vi "Control Page.vi"(8 "?":errorcluster) -> ()   [LabVIEW 2023, in "Vires VTD System Explorer.lvlib"]
uses:
  Vires VTD System Explorer.lvlib
  <vilib>/NI VeriStand/Custom Device API/Custom Device Item Ref.ctl
  <vilib>/NI VeriStand/Custom Device API/Custom Device API.lvlib
panel:
  in  "Header":cluster{"Section Name":string}={"Section Name"="Custom Device Item Settings"}
  in  "Description":string
  in  "Name":string
  in  "Node Ptr":T1 format="%.0x"
  out "error out":errorcluster
  in  "SHDocVw.IWebBrowser2":refnum<k7>(container)
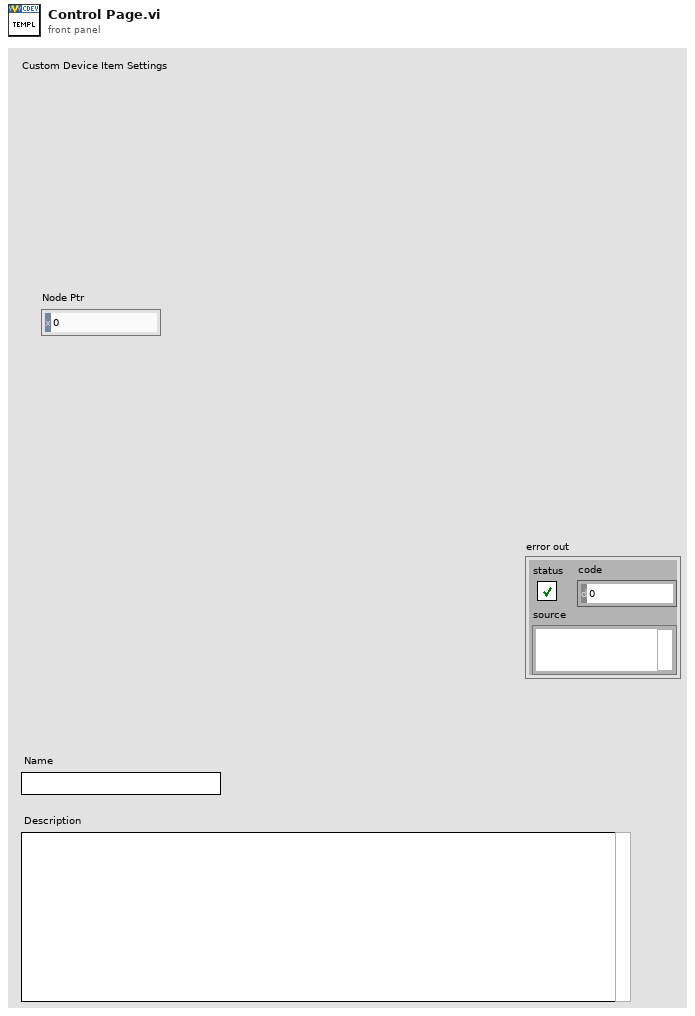
[diagram p1: front panel]
types:
  T1 = typedef "Custom Device API.lvlib/Custom Device Item Ref.ctl" = u64
  T2 = typedef "Custom Device API.lvlib/Custom Device Item Info.ctl" = cluster{"Name":string, "Is Channel":bool, "GUID":string, "Is Waveform":bool}
  T3 = typedef "Custom Device API.lvlib/Custom Device Commands.ctl" = enum16{"Default", "Item renamed", "Shutdown", "Dynamic button pressed"}
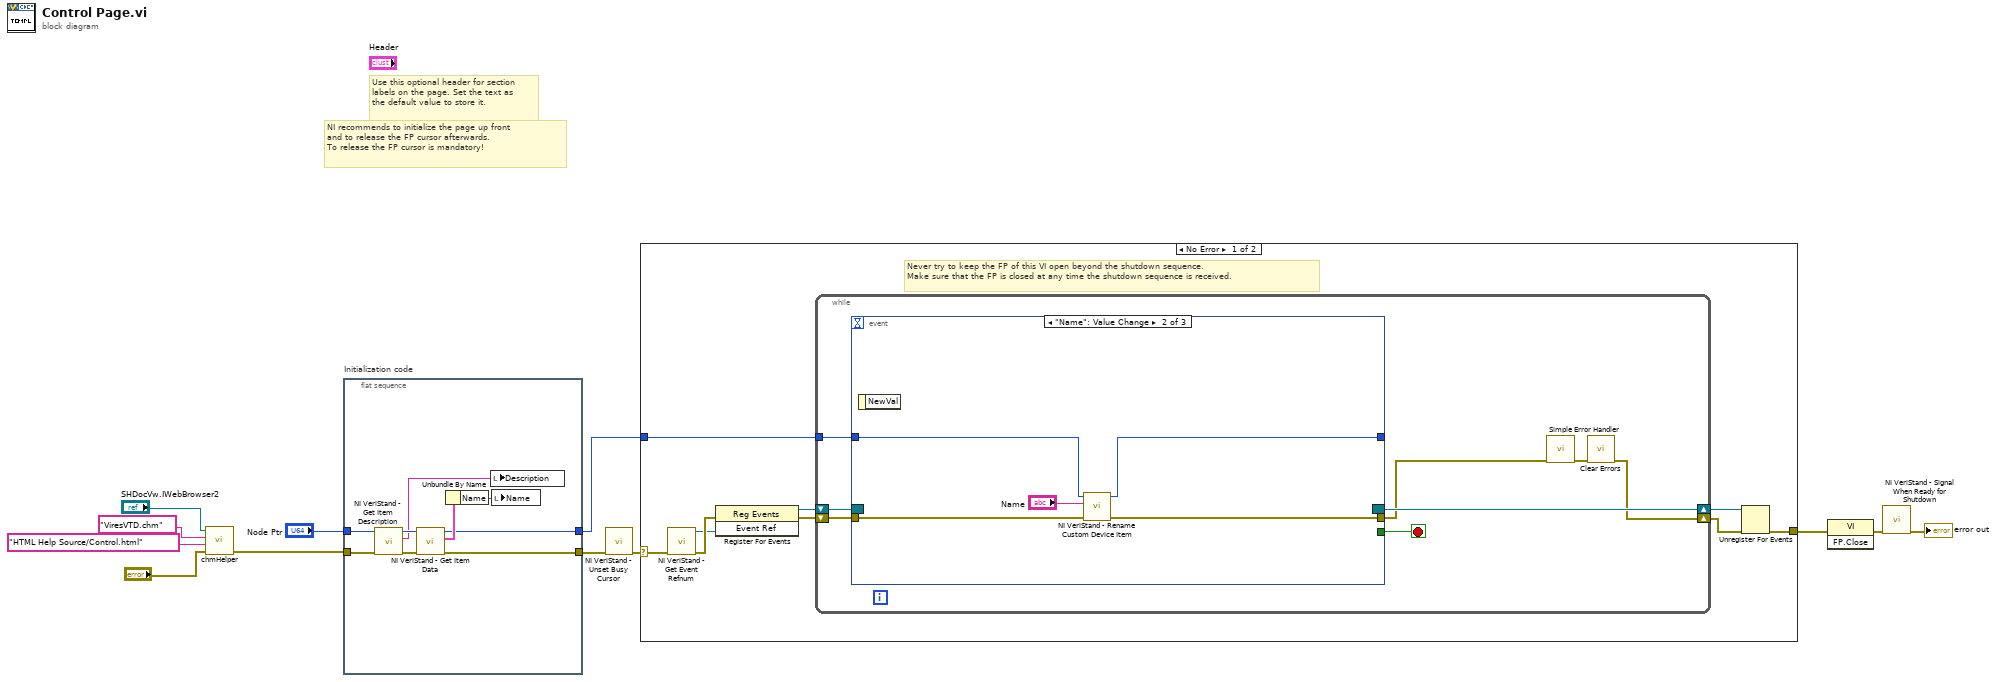
[diagram p0: block diagram]
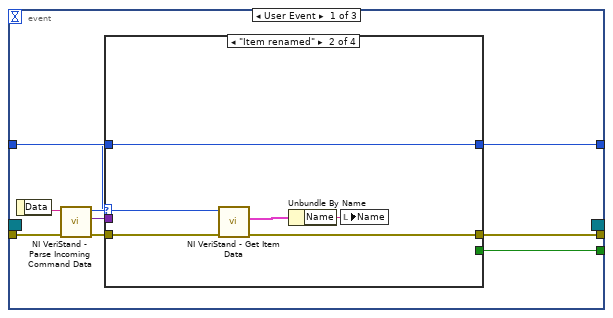
[diagram p2: hidden frame]
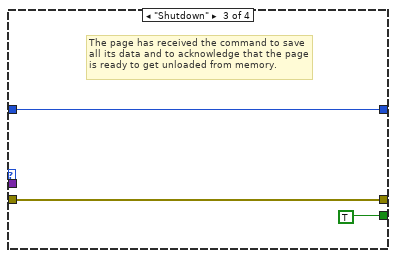
[diagram p4: hidden frame]
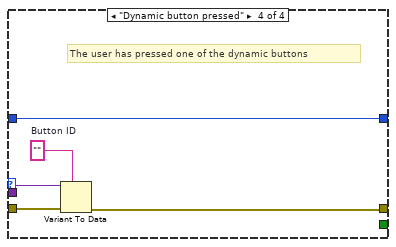
[diagram p5: hidden frame]
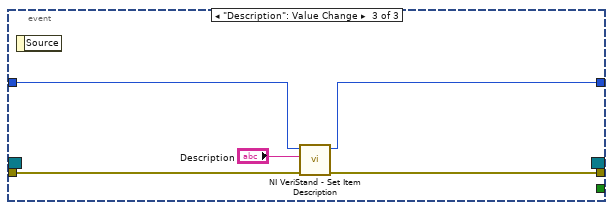
[diagram p6: hidden frame]
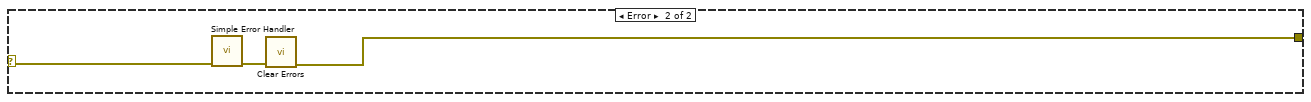
[diagram p7: hidden frame]
diagram:
  # "Use this optional header for section labels on the page. Set the text as the default value to store it."
  # "NI recommends to initialize the page up front\nand to release the FP cursor afterwards.\nTo release the FP cursor is mandatory!"
  n1 = call "chmHelper.vi"("error in (no error)"="?", "HTML File"="HTML Help Source/Control.html", "Main CHM File"="ViresVTD.chm" ("HTML File"), "Automation Refnum in"="SHDocVw.IWebBrowser2") -> ("error out"=w1:errorcluster)  [unwired: 7 in]
  n2 = flat-sequence "Initialization code" {
    tunnel: w1 -> [w20]
    tunnel: "Node Ptr" -> [w19]
    tunnel: [w14] -> w4
    tunnel: [w13] -> w2
    frame #0 {
      n3 = call <vilib>:"NI VeriStand - Get Item Description.vi"("error in (no error)"=w20, "Item Ref in"=w19) -> ("error out"=w17:errorcluster, "Description"=w18:string, "Item Ref out"=w21:T1)  [unwired: 7 out]
      n4 = call <vilib>:"NI VeriStand - Get Item Data.vi"("error in (no error)"=w17, "Item Ref in"=w21) -> ("error out"=w14:errorcluster, "Item Info"=w16:T2, "Item Ref out"=w13:T1)  [unwired: 7 out]
      n5 = Unbundle By Name(w16) -> ("Name"=w15:string)
      n6 = local write "Description"(w18) -> ()
      n7 = local write "Name"(w15) -> ()
    }
  }
  n8 = call <vilib>:"NI VeriStand - Unset Busy Cursor.vi"("error in (no error)"=w4) -> ("error out"=w3:errorcluster)  [unwired: 10 out]
  n9 = case shown="No Error" w3 {
    selector: w3 -> [w22 w75]
    tunnel: [w27 w73] -> w8
    tunnel: w2 -> [w23 _]
    frame No Error {
      # "Never try to keep the FP of this VI open beyond the shutdown sequence.\nMake sure that the FP is closed at any time the shutdown sequence is received."
      n10 = call <vilib>:"NI VeriStand - Get Event Refnum.vi"("error in (no error)"=w22) -> ("error out"=w30:errorcluster, "Event Ref"=w26:refnum<user-event>)  [unwired: 9 out]
      n11 = register-events(error in=w30, w26) -> (reference out=w24:refnum<event-registration>, error out=w25:errorcluster)  [unwired: 1 in]
      n12 = while {
        tunnel: w23 -> [w34]
        shift-right: [w31] -> w28
        shift-left: w25 -> [w37]
        shift-right: [w38] -> w29
        shift-left: w24 -> [w36]
        stop <- w35 stop-if-true
        n13 = event shown="[1] \"Name\": Value Change" {
          selector: w36 -> [_ _ _]
          dyn-events: [_ _ _] -> w38
          timeout: _ -> [_ _ _]
          tunnel: w37 -> [w47 w67 w71]
          tunnel: [w43 _ _] -> w35
          tunnel: [w42 w66 w70] -> w33
          tunnel: w34 -> [w41 w65 w72]
          tunnel: [w39 w63 w68] -> _
          event User Event {
            n14 = event-data() -> ("Data"=w46:string)  [unwired: 1 out]
            n15 = call <vilib>:"NI VeriStand - Parse Incoming Command Data.vi"("error in (no error)"=w47, "Incoming data"=w46) -> ("error out"=w45:errorcluster, "Outgoing data"=w40:variant, "Action"=w44:T3)  [unwired: 7 out]
            n16 = case shown="\"Item renamed\"" w44 {
              tunnel: w45 -> [w49 w54 w56 w62]
              tunnel: [_ _ TRUE _] -> w43
              tunnel: [w49 w52 w56 w59] -> w42
              tunnel: w41 -> [w48 w50 w55 w58]
              tunnel: w40 -> [_ _ _ w61]
              tunnel: [w48 w50 w55 w58] -> w39
              frame "Default", Default {
              }
              frame "Item renamed" {
                n17 = call <vilib>:"NI VeriStand - Get Item Data.vi"("error in (no error)"=w54, "Item Ref in"=w50) -> ("error out"=w52:errorcluster, "Item Info"=w53:T2)  [unwired: 8 out]
                n18 = Unbundle By Name(w53) -> ("Name"=w51:string)
                n19 = local write "Name"(w51) -> ()
              }
              frame "Shutdown" {
                # "The page has received the command to save all its data and to acknowledge that the page is ready to get unloaded from memory."
              }
              frame "Dynamic button pressed" {
                w60 = ""  # Button ID
                # "The user has pressed one of the dynamic buttons"
                n20 = Variant To Data(error in=w62, type=w60, Variant=w61) -> (error out=w59:errorcluster)  [unwired: 1 out]
              }
            }
          }
          event "Name": Value Change {
            n21 = event-data() -> ()  [unwired: 2 out]
            n22 = call <vilib>:"NI VeriStand - Rename Custom Device Item.vi"("error in (no error)"=w67, "New Name"="Name", "Item Ref in"=w65) -> ("error out"=w66:errorcluster, "Item Ref out"=w63:T1)  [unwired: 1 in, 6 out]
          }
          event "Description": Value Change {
            n23 = event-data() -> ()  [unwired: 2 out]
            n24 = call <vilib>:"NI VeriStand - Set Item Description.vi"("error in (no error)"=w71, "Description"="Description", "Item Ref in"=w72) -> ("error out"=w70:errorcluster, "Item Ref out"=w68:T1)  [unwired: 7 out]
          }
        }
        n25 = call <vilib>:"Simple Error Handler.vi"("error in (no error)"=w33) -> ("error out"=w32:errorcluster)  [unwired: 1 in, 7 out]
        n26 = call <vilib>:"Clear Errors.vi"("error in (no error)"=w32) -> ("error out"=w31:errorcluster)  [unwired: 1 in, 5 out]
      }
      n27 = Unregister For Events(event registration refnum=w29, error in=w28) -> (error out=w27:errorcluster)
    }
    frame Error {
      n28 = call <vilib>:"Simple Error Handler.vi"("error in (no error)"=w75) -> ("error out"=w74:errorcluster)  [unwired: 1 in, 7 out]
      n29 = call <vilib>:"Clear Errors.vi"("error in (no error)"=w74) -> ("error out"=w73:errorcluster)  [unwired: 1 in, 5 out]
    }
  }
  n30 = invoke class="VI" method="FP.Close"(error in=w8) -> (error out=w7:errorcluster)  [unwired: 2 in, 2 out]
  n31 = call <vilib>:"NI VeriStand - Signal When Ready for Shutdown.vi"("error in (no error)"=w7) -> ("error out"=→"error out":errorcluster)  [unwired: 10 out]
